vi "Jogosultságok mentés.vi"(8 "error in":errorcluster, 11 "Jogosultság adatok in":T1[](array[typedef])) -> (0 "error out":errorcluster)   [LabVIEW 2014]
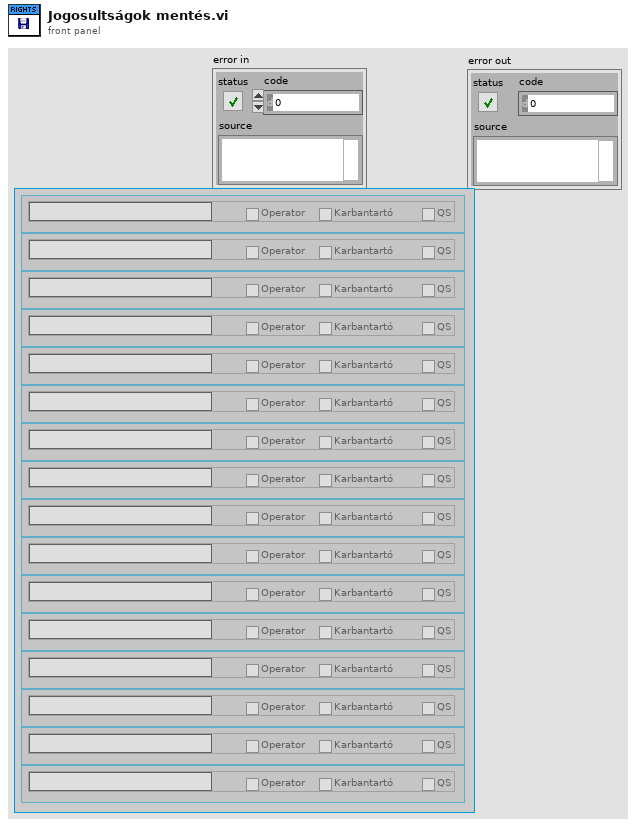
[diagram p1: front panel]
types:
  T1 = typedef "Tab jogosultság.ctl" = cluster{"Tab Name":string, "Operator":bool, "Karbantartó":bool, "QS":bool}
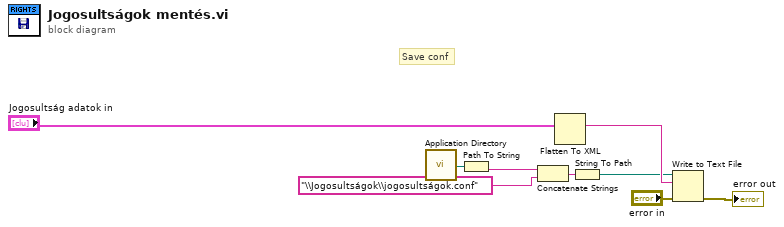
[diagram p0: block diagram]
diagram:
  # "Save conf"
  n1 = call <vilib>:"Application Directory.vi"() -> ("Application Directory"=w8:path)
  n2 = Path To String(path=w8) -> (string=w6:string)
  n3 = Concatenate Strings(w6, "\\Jogosultságok\\jogosultságok.conf" ("prompt (Choose or enter file path)")) -> (w7:string)
  n4 = Flatten To XML(anything="Jogosultság adatok in") -> (xml string=w9:string)
  n5 = String To Path(string=w7) -> (path=w4:path)
  n6 = Write to Text File(file (use dialog)=w4, text=w9, error in="error in") -> (error out=→"error out":errorcluster)  [unwired: 1 in, 2 out]
